vi "Set fan speed.vi"(8 "error in (no error)":errorcluster, 10 "Fan speed":u8, 11 "VISA resource name":refnum<visa-resource-name>) -> (0 "error out":errorcluster, 3 "VISA resource name out":refnum<visa-resource-name>)   [LabVIEW 2023, in "Marlin Instrument Driver.lvlib"]
doc: "Returns the current state of the configured X, Y, Z endstops. Takes into account any 'inverted endstop' settings, so one can confirm that the machine is interpreting the endstops correctly."
uses:
  Marlin Instrument Driver.lvlib
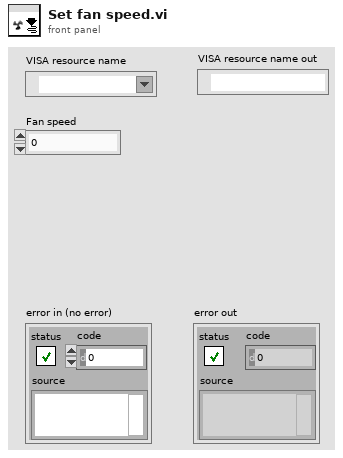
[diagram p1: front panel]
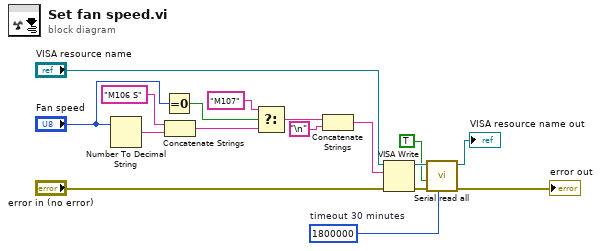
[diagram p0: block diagram]
diagram:
  w10 = u32 1800000  # timeout 30 minutes
  n1 = Number To Decimal String(number="Fan speed") -> (decimal integer string=w8:string)  [unwired: 1 in]
  n2 = Equal To 0?(x="Fan speed") -> (x = 0?=w5:bool)
  n3 = Concatenate Strings("M106 S", w8) -> (w6:string)
  n4 = Select(t="M107", s=w5, f=w6) -> (s? t:f=w3:string)
  n5 = Concatenate Strings(w3, "\n") -> (w1:string)
  n6 = VISA Write(VISA resource name="VISA resource name", write buffer=w1, error in (no error)="error in (no error)") -> (VISA resource name out=w14:refnum<visa-resource-name>, error out=w15:errorcluster)  [unwired: 1 out]
  n7 = call "Serial read all.vi"("timeout (10000ms)"=w10, "error in (no error)"=w15, "Wait for OK"=TRUE, "VISA Refnum in"=w14) -> ("error out"=→"error out":errorcluster, "VISA Refnum out"=→"VISA resource name out":refnum<visa-resource-name>)  [unwired: 4 in, 2 out]
